vi "MOCVD_FrontPanelr.vi"() -> ()   [LabVIEW 2011]
uses:
  low_level_proc/globals.vi
panel:
  in  "Clear Log":bool
  in  "?":enum32{"Vacuum", "Heater/Spinner"}(tab)
  in  "Vac Remote":bool
  in  "Vac Exhaust":bool
  in  "Atm Exhaust":bool
  in  "Set":bool
  in  "Setpoint (C)":dbl
  in  "Heater":bool
  in  "Spinner":bool
  in  "Heater/Spinner Remote":bool
  out "Log":string
  in  "Clear All Relays":bool
  in  "Stop":bool
  in  "?":T1(tab)
  in  "display N2 or H2":bool=TRUE
  in  "N2/H2 Remote":bool
  in  "Set N2 Flow Rate":dbl min=0.0 max=1000.0
  in  "Set H2 Flow Rate":dbl min=0.0 max=1000.0
  out "H2/N2 Actual Flow Rate":dbl
  in  "N2 On":bool
  in  "H2 On":bool
  in  "Set Al Flow Rate":dbl min=0.0 max=100.0
  out "Actual Al Flow Rate":dbl
  in  "Al Remote":bool
  in  "Al Active":bool
  in  "Al Bubbler":bool
  in  "Al Run":bool
  out "GAMFC1":dbl format="%4.2g"
  out "GAMFC2":dbl format="%4.2g"
  out "GAMFC3":i16
  in  "Ga Set  Flow Rate 2 (Bubbler)":dbl min=0.0 max=10.0 format="%4.2f"
  in  "Ga Set Flow Rate 1 (Out)":dbl min=0.0 max=1.0 format="%4.2g"
  in  "Ga Active":bool
  in  "Ga Bubbler":bool
  in  "Ga Run":bool
  in  "Ga H2 Dilute":bool
  in  "Ga Remote":bool
  in  "Ga Set Flow Rate 3 (Vent)":i16 min=0 max=1000
  in  "Set In Flow Rate":dbl min=0.0 max=100.0
  out "Actual In Flow Rate":dbl
  in  "In Remote":bool
  in  "In Active":bool
  in  "In Bubbler":bool
  in  "In Run":bool
  in  "Set P_Gas Flow Rate":dbl min=0.0 max=1000.0
  out "Actual P_Gas Flow Rate":dbl
  in  "P_Gas Remote":bool
  in  "P_Gas Active":bool
  in  "P_Gas In":bool
  in  "P_Gas Run":bool
  in  "P_Gas H2 In":bool
  in  "As Gas Set Flow Rate":dbl min=0.0 max=1000.0
  out "As Gas Actual Flow Rate":dbl
  in  "As Gas Run":bool
  in  "As Gas  H2 In":bool
  in  "As Gas Active":bool
  in  "As Gas In":bool
  in  "As Gas Remote":bool
  in  "Set P_Liq Flow Rate":dbl min=0.0 max=100.0
  out "Actual P_Liq Flow Rate":dbl
  in  "P_Liq Remote":bool
  in  "P_Liq Active":bool
  in  "P_Liq Bubbler":bool
  in  "P_Liq Run":bool
  in  "Set As_Liq Flow Rate":dbl min=0.0 max=100.0
  out "Actual As_Liq Flow Rate":dbl
  in  "As_Liq Remote":bool
  in  "As_Liq Active":bool
  in  "As_Liq Bubbler":bool
  in  "As_Liq Run":bool
  out "Actual Flow Rate 1 (Out)":dbl
  out "Actual Flow Rate 2 (Bubbler)":dbl
  out "Actual Flow Rate 3 (Vent)":dbl
  in  "Fe Set Flow Rate 1 (Out)":dbl min=0.0 max=100.0
  in  "Fe SetFlow Rate 2 (Bubbler)":dbl min=0.0 max=100.0
  in  "Fe Active":bool
  in  "Fe Bubbler":bool
  in  "Fe H2 Dilute":bool
  in  "Fe Run":bool
  in  "Fe Remote":bool
  in  "Fe Set Flow Rate 3 (Vent)":dbl min=0.0 max=100.0
  in  "?":enum32{"P-Dopant", "N-Dopant"}(tab)
  in  "P_Dop Gas Source":bool
  in  "P_Dop H2 Dilute":bool
  in  "P_Dop Run":bool
  in  "P_Dop Bubbler":bool
  in  "P_Dop Active":bool
  in  "Set P Dopant Flow Rate 1":dbl min=0.0 max=100.0
  in  "Set P Dopant Flow Rate 2":dbl min=0.0 max=100.0
  in  "Set P Dopant Flow Rate 3":dbl min=0.0 max=1000.0
  in  "Set P Dopant Flow Rate 4":dbl min=0.0 max=100.0
  in  "P_Dop Remote":bool
  in  "Set N Dopant Flow Rate 1":dbl min=0.0 max=100.0
  in  "Set N Dopant Flow Rate 2":dbl min=0.0 max=100.0
  in  "Set N Dopant Flow Rate 3":dbl min=0.0 max=1000.0
  in  "Set N Dopant Flow Rate 4":dbl min=0.0 max=10.0
  in  "N_Dop Remote":bool
  in  "N_Dop Gas Source":bool
  in  "N_Dop H2 Dilute":bool
  in  "N_Dop Run":bool
  in  "N_Dop Active":bool
  in  "N_Dop Bubbler":bool
  out "Actual NP Dopant Flow Rate 1":dbl
  out "Actual NP Dopant Flow Rate 2, 4":dbl
  out "Actual N Dopant Flow Rate 3":dbl
  in  "Display N or P":bool
  in  "6940B GPIB Address":string="23"
  # "0-10000 sscm"
  # "0-10000 sscm"
  # "Display:"
  # "N2"
  # "H2"
  # "100 sscm"
  # "10 sscm"
  # "10 sscm"
  # "1000 sscm"
  # "100 sscm"
  # "100 sscm"
  # "10 sscm"
  # "100 sscm"
  # "100 sscm"
  # "100 sscm"
  # "100 sscm"
  # "1000 sscm"
  # "100 sscm"
  # "100 sscm"
  # "1000 sscm"
  # "100 sscm"
  # "100 sscm"
  # "100 sscm"
  # "1000 sscm"
  # "10 sscm"
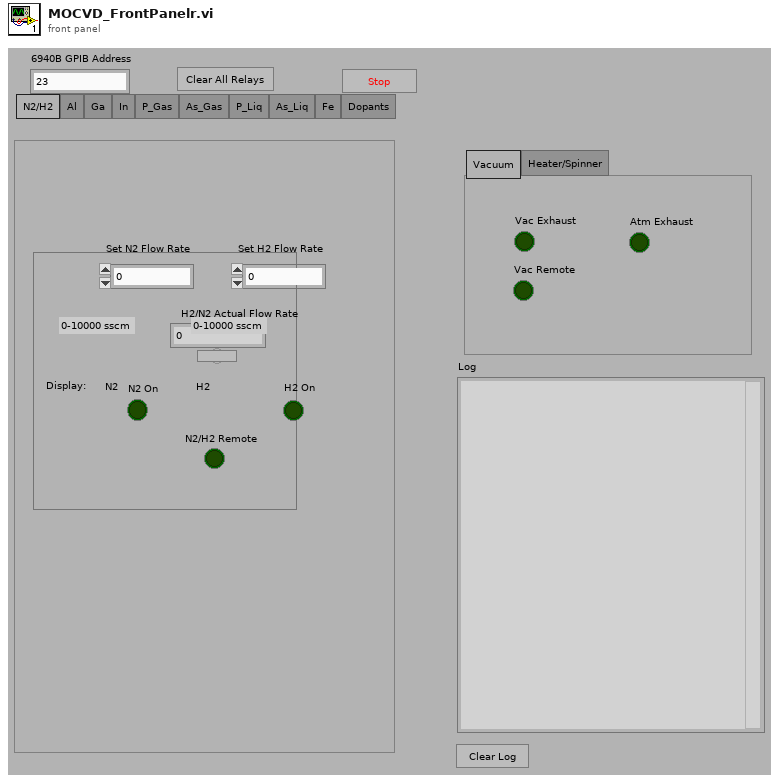
[diagram p1: front panel]
types:
  T1 = enum32{"N2/H2", "Al", "Ga", "In", "P_Gas", "As_Gas", "P_Liq", "As_Liq", "Fe", "Dopants"}
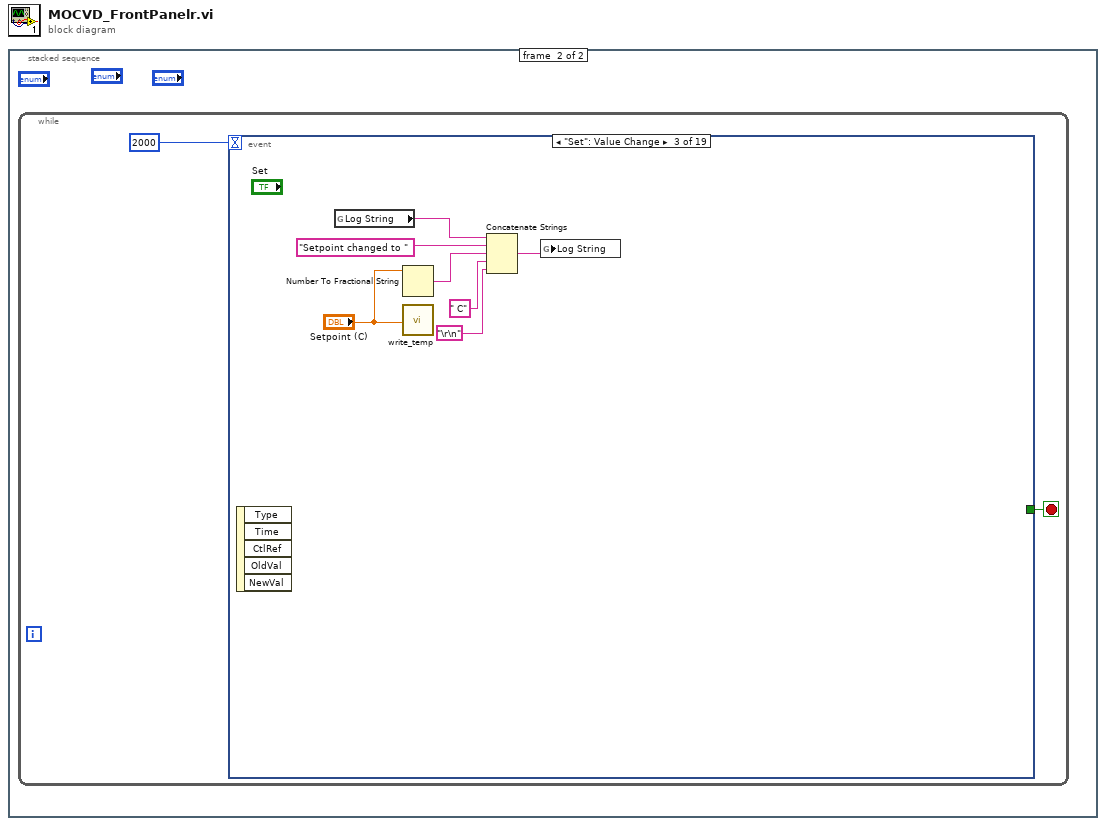
[diagram p0: block diagram]
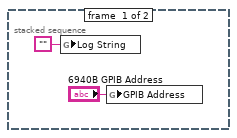
[diagram p2: hidden frame]
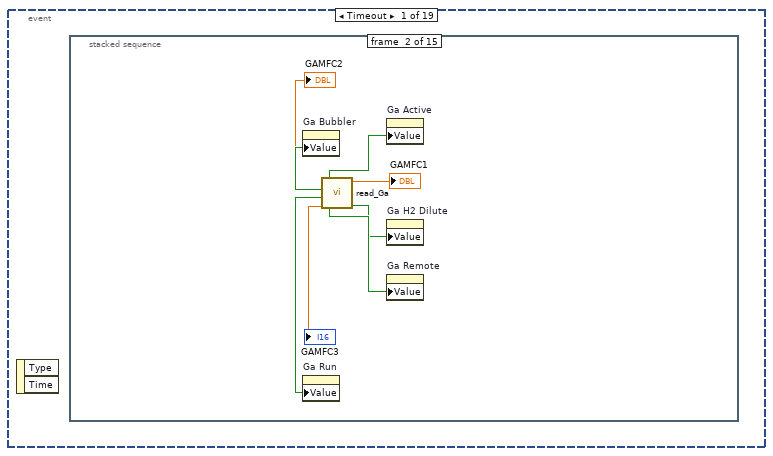
[diagram p3: hidden frame]
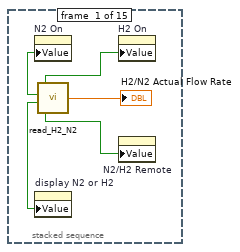
[diagram p4: hidden frame]
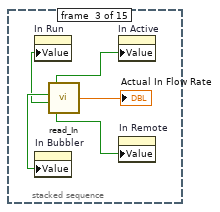
[diagram p5: hidden frame]
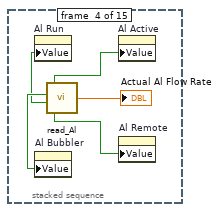
[diagram p6: hidden frame]
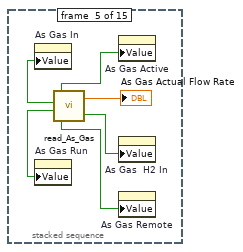
[diagram p7: hidden frame]
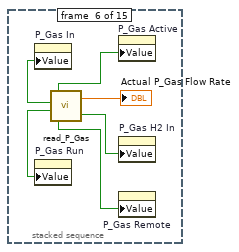
[diagram p8: hidden frame]
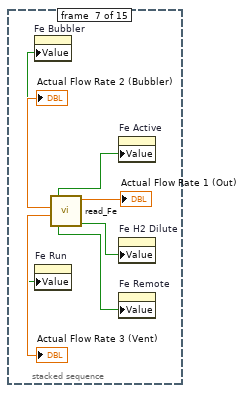
[diagram p9: hidden frame]
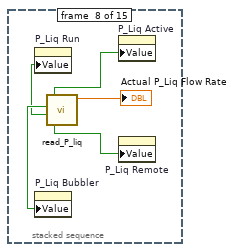
[diagram p10: hidden frame]
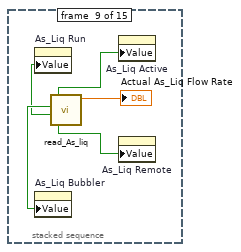
[diagram p11: hidden frame]
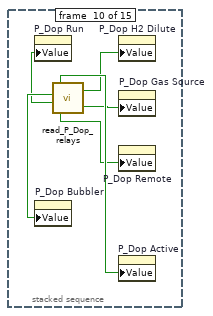
[diagram p12: hidden frame]
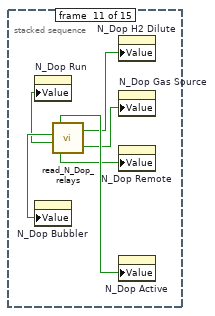
[diagram p13: hidden frame]
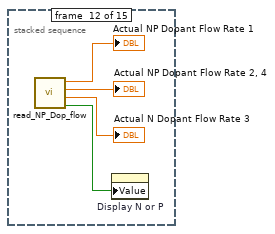
[diagram p14: hidden frame]
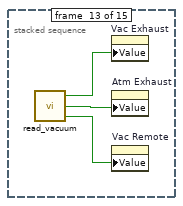
[diagram p15: hidden frame]
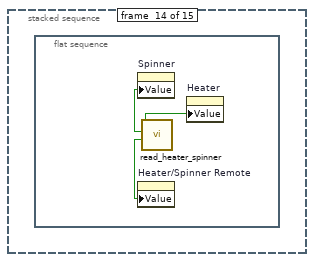
[diagram p16: hidden frame]
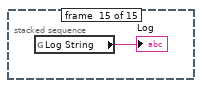
[diagram p17: hidden frame]
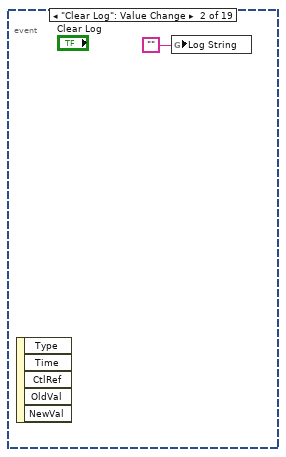
[diagram p18: hidden frame]
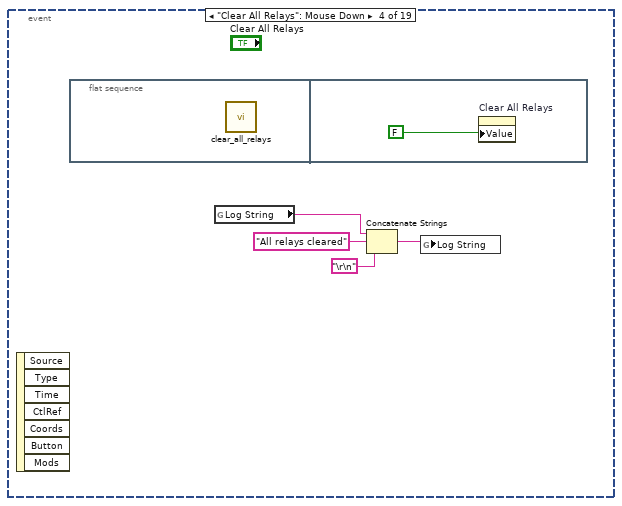
[diagram p19: hidden frame]
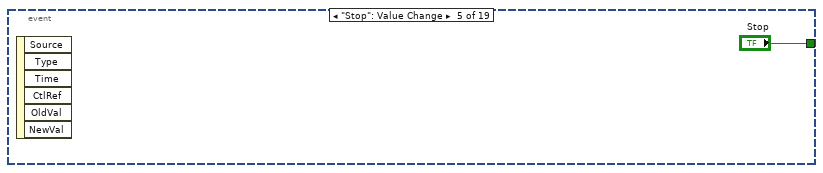
[diagram p20: hidden frame]
diagram:
  n1 = stacked-sequence {
    frame #0 {
      n2 = global write "globals.vi" "Log String"("") -> ()
      n3 = global write "globals.vi" "GPIB Address"("6940B GPIB Address") -> ()
    }
    frame #1 {
      n4 = while {
        stop <- w4 stop-if-true
        n5 = event shown="[2] \"Set\": Value Change" {
          selector: _ -> [_ _ _ _ _ _ _ _ _ _ _ _ _ _ _ _ _ _ _]
          dyn-events: _ -> [_ _ _ _ _ _ _ _ _ _ _ _ _ _ _ _ _ _ _]
          timeout: 2000 -> [_ _ _ _ _ _ _ _ _ _ _ _ _ _ _ _ _ _ _]
          tunnel: [_ _ _ _ "Stop" _ _ _ _ _ _ _ _ _ _ _ _ _ _] -> w4
          event Timeout {
            n6 = event-data() -> ()  [unwired: 3 out]
            n7 = stacked-sequence {
              frame #0 {
                n8 = call "read_H2_N2.vi"() -> ("H2N2 Flow Rate"=→"H2/N2 Actual Flow Rate":dbl, "H2N2 Remote"=w9:bool, "Display H2N2"=w8:bool, "N2 Active"=w7:bool, "H2 Active"=w6:bool)
                n9 = property on="N2 On" class="Bool (strict)"("Value"=w7) -> ()  [unwired: 2 in, 2 out]
                n10 = property on="display N2 or H2" class="Bool (strict)"("Value"=w8) -> ()  [unwired: 2 in, 2 out]
                n11 = property on="H2 On" class="Bool (strict)"("Value"=w6) -> ()  [unwired: 2 in, 2 out]
                n12 = property on="N2/H2 Remote" class="Bool (strict)"("Value"=w9) -> ()  [unwired: 2 in, 2 out]
              }
              frame #1 {
                n13 = call "read_Ga.vi"() -> ("H2 Dilute"=w13:bool, "GAMFC3"=→"GAMFC3":dbl, "GAMFC2"=→"GAMFC2":dbl, "GAMFC1"=→"GAMFC1":dbl, "Ga Remote"=w16:bool, "Ga Run"=w17:bool, "Ga Bubbler"=w14:bool, "Ga Active"=w15:bool)
                n14 = property on="Ga Bubbler" class="Bool (strict)"("Value"=w14) -> ()  [unwired: 2 in, 2 out]
                n15 = property on="Ga Run" class="Bool (strict)"("Value"=w17) -> ()  [unwired: 2 in, 2 out]
                n16 = property on="Ga Active" class="Bool (strict)"("Value"=w15) -> ()  [unwired: 2 in, 2 out]
                n17 = property on="Ga H2 Dilute" class="Bool (strict)"("Value"=w13) -> ()  [unwired: 2 in, 2 out]
                n18 = property on="Ga Remote" class="Bool (strict)"("Value"=w16) -> ()  [unwired: 2 in, 2 out]
              }
              frame #2 {
                n19 = call "read_In.vi"() -> ("Actual In Flow Rate"=→"Actual In Flow Rate":dbl, "In Remote"=w19:bool, "In Run"=w18:bool, "In Bubbler"=w20:bool, "In Active"=w21:bool)
                n20 = property on="In Run" class="Bool (strict)"("Value"=w18) -> ()  [unwired: 2 in, 2 out]
                n21 = property on="In Bubbler" class="Bool (strict)"("Value"=w20) -> ()  [unwired: 2 in, 2 out]
                n22 = property on="In Active" class="Bool (strict)"("Value"=w21) -> ()  [unwired: 2 in, 2 out]
                n23 = property on="In Remote" class="Bool (strict)"("Value"=w19) -> ()  [unwired: 2 in, 2 out]
              }
              frame #3 {
                n24 = call "read_Al.vi"() -> ("Actual Al Flow Rate"=→"Actual Al Flow Rate":dbl, "Al Remote"=w23:bool, "Al Run"=w25:bool, "Al Bubbler"=w26:bool, "Al Active"=w27:bool)
                n25 = property on="Al Run" class="Bool (strict)"("Value"=w25) -> ()  [unwired: 2 in, 2 out]
                n26 = property on="Al Bubbler" class="Bool (strict)"("Value"=w26) -> ()  [unwired: 2 in, 2 out]
                n27 = property on="Al Active" class="Bool (strict)"("Value"=w27) -> ()  [unwired: 2 in, 2 out]
                n28 = property on="Al Remote" class="Bool (strict)"("Value"=w23) -> ()  [unwired: 2 in, 2 out]
              }
              frame #4 {
                n29 = call "read_As_Gas.vi"() -> ("As Gas H2 In"=w28:bool, "As Gas Actual Flow Rate"=→"As Gas Actual Flow Rate":dbl, "As Gas Remote"=w32:bool, "As Gas Run"=w31:bool, "As Gas In"=w30:bool, "As Gas Active"=w29:bool)
                n30 = property on="As Gas In" class="Bool (strict)"("Value"=w30) -> ()  [unwired: 2 in, 2 out]
                n31 = property on="As Gas Run" class="Bool (strict)"("Value"=w31) -> ()  [unwired: 2 in, 2 out]
                n32 = property on="As Gas Active" class="Bool (strict)"("Value"=w29) -> ()  [unwired: 2 in, 2 out]
                n33 = property on="As Gas  H2 In" class="Bool (strict)"("Value"=w28) -> ()  [unwired: 2 in, 2 out]
                n34 = property on="As Gas Remote" class="Bool (strict)"("Value"=w32) -> ()  [unwired: 2 in, 2 out]
              }
              frame #5 {
                n35 = call "read_P_Gas.vi"() -> ("P Gas H2 In"=w34:bool, "P Gas Actual Flow Rate"=→"Actual P_Gas Flow Rate":dbl, "P Gas Remote"=w38:bool, "P Gas Run"=w37:bool, "P Gas In"=w36:bool, "P Gas Active"=w35:bool)
                n36 = property on="P_Gas In" class="Bool (strict)"("Value"=w36) -> ()  [unwired: 2 in, 2 out]
                n37 = property on="P_Gas Run" class="Bool (strict)"("Value"=w37) -> ()  [unwired: 2 in, 2 out]
                n38 = property on="P_Gas Active" class="Bool (strict)"("Value"=w35) -> ()  [unwired: 2 in, 2 out]
                n39 = property on="P_Gas H2 In" class="Bool (strict)"("Value"=w34) -> ()  [unwired: 2 in, 2 out]
                n40 = property on="P_Gas Remote" class="Bool (strict)"("Value"=w38) -> ()  [unwired: 2 in, 2 out]
              }
              frame #6 {
                n41 = call "read_Fe.vi"() -> ("Fe H2 Dilute"=w44:bool, "Actual Fe Flow Rate 3 (Vent)"=→"Actual Flow Rate 3 (Vent)":dbl, "Actual Fe Flow Rate2 (Bubbler)"=→"Actual Flow Rate 2 (Bubbler)":dbl, "Actual Fe Flow Rate1  (Out)"=→"Actual Flow Rate 1 (Out)":dbl, "Fe Remote"=w43:bool, "Fe Run"=w42:bool, "Fe Bubbler"=w41:bool, "Fe Active"=w40:bool)
                n42 = property on="Fe Bubbler" class="Bool (strict)"("Value"=w41) -> ()  [unwired: 2 in, 2 out]
                n43 = property on="Fe Run" class="Bool (strict)"("Value"=w42) -> ()  [unwired: 2 in, 2 out]
                n44 = property on="Fe Active" class="Bool (strict)"("Value"=w40) -> ()  [unwired: 2 in, 2 out]
                n45 = property on="Fe H2 Dilute" class="Bool (strict)"("Value"=w44) -> ()  [unwired: 2 in, 2 out]
                n46 = property on="Fe Remote" class="Bool (strict)"("Value"=w43) -> ()  [unwired: 2 in, 2 out]
              }
              frame #7 {
                n47 = call "read_P_liq.vi"() -> ("Actual P liq Flow Rate"=→"Actual P_Liq Flow Rate":dbl, "P liq Remote"=w49:bool, "P liq Run"=w48:bool, "P liq Bubbler"=w51:bool, "P liq Active"=w50:bool)  [unwired: 3 out]
                n48 = property on="P_Liq Run" class="Bool (strict)"("Value"=w48) -> ()  [unwired: 2 in, 2 out]
                n49 = property on="P_Liq Bubbler" class="Bool (strict)"("Value"=w51) -> ()  [unwired: 2 in, 2 out]
                n50 = property on="P_Liq Active" class="Bool (strict)"("Value"=w50) -> ()  [unwired: 2 in, 2 out]
                n51 = property on="P_Liq Remote" class="Bool (strict)"("Value"=w49) -> ()  [unwired: 2 in, 2 out]
              }
              frame #8 {
                n52 = call "read_As_liq.vi"() -> ("Actual As liq Flow Rate"=→"Actual As_Liq Flow Rate":dbl, "As liq Remote"=w53:bool, "As liq Run"=w54:bool, "As liq Bubbler"=w55:bool, "As liq Active"=w56:bool)  [unwired: 3 out]
                n53 = property on="As_Liq Run" class="Bool (strict)"("Value"=w54) -> ()  [unwired: 2 in, 2 out]
                n54 = property on="As_Liq Bubbler" class="Bool (strict)"("Value"=w55) -> ()  [unwired: 2 in, 2 out]
                n55 = property on="As_Liq Active" class="Bool (strict)"("Value"=w56) -> ()  [unwired: 2 in, 2 out]
                n56 = property on="As_Liq Remote" class="Bool (strict)"("Value"=w53) -> ()  [unwired: 2 in, 2 out]
              }
              frame #9 {
                n57 = call "read_P_Dop_relays.vi"() -> ("P_Dop Gas Source"=w60:bool, "P_Dop H2 Dilute"=w61:bool, "P_Dop Remote"=w58:bool, "P_Dop Run"=w59:bool, "P_Dop Bubbler"=w62:bool, "P_Dop Active"=w63:bool)
                n58 = property on="P_Dop Run" class="Bool (strict)"("Value"=w59) -> ()  [unwired: 2 in, 2 out]
                n59 = property on="P_Dop Bubbler" class="Bool (strict)"("Value"=w62) -> ()  [unwired: 2 in, 2 out]
                n60 = property on="P_Dop H2 Dilute" class="Bool (strict)"("Value"=w61) -> ()  [unwired: 2 in, 2 out]
                n61 = property on="P_Dop Gas Source" class="Bool (strict)"("Value"=w60) -> ()  [unwired: 2 in, 2 out]
                n62 = property on="P_Dop Remote" class="Bool (strict)"("Value"=w58) -> ()  [unwired: 2 in, 2 out]
                n63 = property on="P_Dop Active" class="Bool (strict)"("Value"=w63) -> ()  [unwired: 2 in, 2 out]
              }
              frame #10 {
                n64 = call "read_N_Dop_relays.vi"() -> ("N_Dop Gas Source"=w64:bool, "N_Dop H2 Dilute"=w65:bool, "N_Dop Remote"=w66:bool, "N_Dop Run"=w67:bool, "N_Dop Bubbler"=w68:bool, "N_Dop Active"=w69:bool)
                n65 = property on="N_Dop Run" class="Bool (strict)"("Value"=w67) -> ()  [unwired: 2 in, 2 out]
                n66 = property on="N_Dop Bubbler" class="Bool (strict)"("Value"=w68) -> ()  [unwired: 2 in, 2 out]
                n67 = property on="N_Dop H2 Dilute" class="Bool (strict)"("Value"=w65) -> ()  [unwired: 2 in, 2 out]
                n68 = property on="N_Dop Gas Source" class="Bool (strict)"("Value"=w64) -> ()  [unwired: 2 in, 2 out]
                n69 = property on="N_Dop Remote" class="Bool (strict)"("Value"=w66) -> ()  [unwired: 2 in, 2 out]
                n70 = property on="N_Dop Active" class="Bool (strict)"("Value"=w69) -> ()  [unwired: 2 in, 2 out]
              }
              frame #11 {
                n71 = call "read_NP_Dop_flow.vi"() -> ("N/P Dopant DA Switch"=w73:bool, "N/P_Dop Flow 3"=→"Actual N Dopant Flow Rate 3":dbl, "N/P_Dop Flow 2 or 4"=→"Actual NP Dopant Flow Rate 2, 4":dbl, "N/P_Dop Flow 1"=→"Actual NP Dopant Flow Rate 1":dbl)
                n72 = property on="Display N or P" class="Bool (strict)"("Value"=w73) -> ()  [unwired: 2 in, 2 out]
              }
              frame #12 {
                n73 = call "read_vacuum.vi"() -> ("Vac Remote"=w76:bool, "Atm Exhaust"=w75:bool, "Vac Exhaust"=w74:bool)
                n74 = property on="Vac Exhaust" class="Bool (strict)"("Value"=w74) -> ()  [unwired: 2 in, 2 out]
                n75 = property on="Atm Exhaust" class="Bool (strict)"("Value"=w75) -> ()  [unwired: 2 in, 2 out]
                n76 = property on="Vac Remote" class="Bool (strict)"("Value"=w76) -> ()  [unwired: 2 in, 2 out]
              }
              frame #13 {
                n77 = flat-sequence {
                  frame #0 {
                    n78 = call "read_heater_spinner.vi"() -> ("Heater/Spinner Remote"=w77:bool, "Spinner"=w78:bool, "Heater"=w79:bool)  [unwired: 7 out]
                    n79 = property on="Spinner" class="Bool (strict)"("Value"=w78) -> ()  [unwired: 2 in, 2 out]
                    n80 = property on="Heater/Spinner Remote" class="Bool (strict)"("Value"=w77) -> ()  [unwired: 2 in, 2 out]
                    n81 = property on="Heater" class="Bool (strict)"("Value"=w79) -> ()  [unwired: 2 in, 2 out]
                  }
                }
              }
              frame #14 {
                n82 = global read "globals.vi" "Log String"() -> (→"Log":string)
              }
            }
          }
          event "Clear Log": Value Change {
            n83 = event-data() -> ()  [unwired: 6 out]
            n84 = global write "globals.vi" "Log String"("") -> ()
          }
          event "Set": Value Change {
            n85 = event-data() -> ()  [unwired: 6 out]
            n86 = global read "globals.vi" "Log String"() -> (w87:string)
            n87 = Number To Fractional String(number="Setpoint (C)") -> (F-format string=w86:string)  [unwired: 3 in]
            n88 = call "write_temp.vi"("Temperature (C)"="Setpoint (C)") -> ()  [unwired: 1 out]
            n89 = Concatenate Strings(w87, "Setpoint changed to " ("string"), w86, " C" ("string"), "\r\n") -> (w88:string)
            n90 = global write "globals.vi" "Log String"(w88) -> ()
          }
          event "Clear All Relays": Mouse Down {
            n91 = event-data() -> ()  [unwired: 8 out]
            n92 = flat-sequence {
              frame #0 {
                n93 = call "clear_all_relays.vi"() -> ()  [unwired: 2 out]
              }
              frame #1 {
                n94 = property on="Clear All Relays" class="Bool (strict)"("Value"=FALSE ("Clear All Relays")) -> ()  [unwired: 2 in, 2 out]
              }
            }
            n95 = global read "globals.vi" "Log String"() -> (w91:string)
            n96 = Concatenate Strings(w91, "All relays cleared" ("string"), "\r\n") -> (w92:string)
            n97 = global write "globals.vi" "Log String"(w92) -> ()
          }
          event "Stop": Value Change {
            n98 = event-data() -> ()  [unwired: 7 out]
          }
          event "N2/H2 Remote", "display N2 or H2", "N2 On", "H2 On", "Set N2 Flow Rate", "Set H2 Flow Rate": Value Change {
            n99 = event-data() -> ()  [unwired: 7 out]
            n100 = call "set_N2.vi"("Manifold N2 Flow"="Set N2 Flow Rate", "Display H2 or N2"="display N2 or H2", "N2 Active"="N2 On", "H2N2 Remote"="N2/H2 Remote") -> ()  [unwired: 2 out]
            n101 = call "set_H2.vi"("Manifold H2 Flow"="Set H2 Flow Rate", "Display H2 or N2"="display N2 or H2", "H2 Active"="H2 On", "H2N2 Remote"="N2/H2 Remote") -> ()  [unwired: 2 in]
            n102 = global read "globals.vi" "Log String"() -> (w118:string)
            n103 = Number To Fractional String(number="Set N2 Flow Rate") -> (F-format string=w104:string)  [unwired: 3 in]
            n104 = Number To Fractional String(number="Set H2 Flow Rate") -> (F-format string=w100:string)  [unwired: 3 in]
            n105 = Select(t="N2 On ", s="N2 On", f="") -> (s? t:f=w114:string)
            n106 = Select(t="H2 On ", s="H2 On", f="") -> (s? t:f=w110:string)
            n107 = Select(t="N2/H2 Remote ", s="N2/H2 Remote", f="") -> (s? t:f=w106:string)
            n108 = Concatenate Strings("N2 Rate " ("string"), w104, " " ("string")) -> (w101:string)
            n109 = Concatenate Strings("H2 Rate " ("string"), w100, " " ("string")) -> (w96:string)
            n110 = Concatenate Strings(w118, w114, w110, w106, w101, w96, "\r\n") -> (w119:string)
            n111 = global write "globals.vi" "Log String"(w119) -> ()
          }
          event "In Remote", "In Active", "In Bubbler", "In Run", "Set In Flow Rate": Value Change {
            n112 = event-data() -> ()  [unwired: 7 out]
            n113 = call "set_In.vi"("Indium Flow"="Set In Flow Rate", "In Remote"="In Remote", "In Run"="In Run", "In Bubbler"="In Bubbler", "In Active"="In Active") -> ()  [unwired: 5 out]
            n114 = Number To Fractional String(number="Set In Flow Rate") -> (F-format string=w143:string)  [unwired: 3 in]
            n115 = Concatenate Strings("In Rate " ("string"), w143, " " ("string")) -> (w139:string)
            n116 = Select(t="In Active ", s="In Active", f="") -> (s? t:f=w126:string)
            n117 = Select(t="In Bubbler ", s="In Bubbler", f="") -> (s? t:f=w125:string)
            n118 = Select(t="In Run ", s="In Run", f="") -> (s? t:f=w124:string)
            n119 = Select(t="In Remote ", s="In Remote", f="") -> (s? t:f=w123:string)
            n120 = global read "globals.vi" "Log String"() -> (w140:string)
            n121 = Concatenate Strings(w140, w139, w126, w125, w124, w123, "\r\n") -> (w122:string)
            n122 = global write "globals.vi" "Log String"(w122) -> ()
          }
          event "Al Remote", "Al Active", "Al Bubbler", "Al Run", "Set Al Flow Rate": Value Change {
            n123 = event-data() -> ()  [unwired: 7 out]
            n124 = call "set_Al.vi"("Aluminum Flow"="Set Al Flow Rate", "Al Remote"="Al Remote", "Al Run"="Al Run", "Al Bubbler"="Al Bubbler", "Al Active"="Al Active") -> ()  [unwired: 5 out]
            n125 = Number To Fractional String(number="Set Al Flow Rate") -> (F-format string=w167:string)  [unwired: 3 in]
            n126 = Concatenate Strings("Al Rate " ("string"), w167, " " ("string")) -> (w151:string)
            n127 = Select(t="Al Active ", s="Al Active", f="") -> (s? t:f=w150:string)
            n128 = Select(t="Al Bubbler ", s="Al Bubbler", f="") -> (s? t:f=w149:string)
            n129 = Select(t="Al Run ", s="Al Run", f="") -> (s? t:f=w148:string)
            n130 = Select(t="Al Remote ", s="Al Remote", f="") -> (s? t:f=w147:string)
            n131 = global read "globals.vi" "Log String"() -> (w152:string)
            n132 = Concatenate Strings(w152, w151, w150, w149, w148, w147, "\r\n") -> (w145:string)
            n133 = global write "globals.vi" "Log String"(w145) -> ()
          }
          event "P_Liq Remote", "P_Liq Active", "P_Liq Bubbler", "P_Liq Run", "Set P_Liq Flow Rate": Value Change {
            n134 = event-data() -> ()  [unwired: 7 out]
            n135 = call "set_P_Liq.vi"("P_Liq Flow"="Set P_Liq Flow Rate", "P_Liq Remote"="P_Liq Remote", "P_Liq Run"="P_Liq Run", "P_Liq Bubbler"="P_Liq Bubbler", "P_Liq Active"="P_Liq Active") -> ()  [unwired: 7 out]
            n136 = Number To Fractional String(number="Set P_Liq Flow Rate") -> (F-format string=w190:string)  [unwired: 3 in]
            n137 = Concatenate Strings("P_Liq Rate " ("string"), w190, " " ("string")) -> (w187:string)
            n138 = global read "globals.vi" "Log String"() -> (w188:string)
            n139 = Select(t="P_Liq Active ", s="P_Liq Active", f="") -> (s? t:f=w173:string)
            n140 = Select(t="P_Liq Bubbler ", s="P_Liq Bubbler", f="") -> (s? t:f=w172:string)
            n141 = Select(t="P_Liq Run ", s="P_Liq Run", f="") -> (s? t:f=w171:string)
            n142 = Select(t="P_Liq Remote ", s="P_Liq Remote", f="") -> (s? t:f=w170:string)
            n143 = Concatenate Strings(w188, w187, w173, w172, w171, w170, "\r\n") -> (w186:string)
            n144 = global write "globals.vi" "Log String"(w186) -> ()
          }
          event "As_Liq Remote", "As_Liq Active", "As_Liq Bubbler", "As_Liq Run", "Set As_Liq Flow Rate": Value Change {
            n145 = event-data() -> ()  [unwired: 7 out]
            n146 = call "set_As_Liq.vi"("As_Liq Flow"="Set As_Liq Flow Rate", "As_Liq Remote"="As_Liq Remote", "As_Liq Run"="As_Liq Run", "As_Liq Bubbler"="As_Liq Bubbler", "As_Liq Active"="As_Liq Active") -> ()  [unwired: 7 out]
            n147 = Number To Fractional String(number="Set As_Liq Flow Rate") -> (F-format string=w214:string)  [unwired: 3 in]
            n148 = Concatenate Strings("As_Liq Rate " ("string"), w214, " " ("string")) -> (w199:string)
            n149 = Select(t="As_Liq Active ", s="As_Liq Active", f="") -> (s? t:f=w198:string)
            n150 = Select(t="As_Liq Bubbler ", s="As_Liq Bubbler", f="") -> (s? t:f=w197:string)
            n151 = Select(t="As_Liq Run ", s="As_Liq Run", f="") -> (s? t:f=w196:string)
            n152 = Select(t="As_Liq Remote ", s="As_Liq Remote", f="") -> (s? t:f=w195:string)
            n153 = global read "globals.vi" "Log String"() -> (w200:string)
            n154 = Concatenate Strings(w200, w199, w198, w197, w196, w195, "\r\n") -> (w193:string)
            n155 = global write "globals.vi" "Log String"(w193) -> ()
          }
          event "P_Gas Remote", "P_Gas Active", "P_Gas In", "P_Gas Run", "P_Gas H2 In", "Set P_Gas Flow Rate": Value Change {
            n156 = event-data() -> ()  [unwired: 7 out]
            n157 = call "set_P_gas.vi"("P_Gas Active"="P_Gas Active", "P_Gas Flow"="Set P_Gas Flow Rate", "P_Gas In"="P_Gas In", "P_Gas H2 In"="P_Gas H2 In", "P_Gas Run"="P_Gas Run", "P_Gas Remote"="P_Gas Remote") -> ()  [unwired: 10 out]
            n158 = Number To Fractional String(number="Set P_Gas Flow Rate") -> (F-format string=w242:string)  [unwired: 3 in]
            n159 = Concatenate Strings("P_Gas Rate " ("string"), w242, " " ("string")) -> (w224:string)
            n160 = Select(t="P_Gas Active ", s="P_Gas Active", f="") -> (s? t:f=w223:string)
            n161 = Select(t="P_Gas In ", s="P_Gas In", f="") -> (s? t:f=w222:string)
            n162 = Select(t="P_Gas H2 In ", s="P_Gas H2 In", f="") -> (s? t:f=w221:string)
            n163 = Select(t="P_Gas Remote ", s="P_Gas Remote", f="") -> (s? t:f=w219:string)
            n164 = Select(t="P_Gas Run ", s="P_Gas Run", f="") -> (s? t:f=w220:string)
            n165 = global read "globals.vi" "Log String"() -> (w225:string)
            n166 = Concatenate Strings(w225, w224, w223, w222, w221, w220, w219, "\r\n") -> (w217:string)
            n167 = global write "globals.vi" "Log String"(w217) -> ()
          }
          event "As Gas Remote", "As Gas Run", "As Gas  H2 In", "As Gas In", "As Gas Active", "As Gas Set Flow Rate": Value Change {
            n168 = event-data() -> ()  [unwired: 7 out]
            n169 = call "set_As_gas.vi"("As_Gas Active"="As Gas Active", "As_Gas Flow"="As Gas Set Flow Rate", "As_Gas In"="As Gas In", "As_Gas H2"="As Gas  H2 In", "As_Gas Run"="As Gas Run", "As_Gas Remote"="As Gas Remote") -> ()  [unwired: 10 out]
            n170 = Number To Fractional String(number="As Gas Set Flow Rate") -> (F-format string=w271:string)  [unwired: 3 in]
            n171 = Concatenate Strings("As Gas Rate " ("string"), w271, " " ("string")) -> (w251:string)
            n172 = Select(t="As Gas In ", s="As Gas In", f="") -> (s? t:f=w249:string)
            n173 = Select(t="As Gas Active ", s="As Gas Active", f="") -> (s? t:f=w250:string)
            n174 = Select(t="As Gas H2 In ", s="As Gas  H2 In", f="") -> (s? t:f=w248:string)
            n175 = Select(t="As Gas Run ", s="As Gas Run", f="") -> (s? t:f=w247:string)
            n176 = Select(t="As Gas Remote ", s="As Gas Remote", f="") -> (s? t:f=w246:string)
            n177 = global read "globals.vi" "Log String"() -> (w253:string)
            n178 = Concatenate Strings(w253, w251, w250, w249, w248, w247, w246, "\r\n") -> (w252:string)
            n179 = global write "globals.vi" "Log String"(w252) -> ()
          }
          event "Ga Active", "Ga Bubbler", "Ga Run", "Ga Set Flow Rate 1 (Out)", "Ga Set  Flow Rate 2 (Bubbler)", "Ga Set Flow Rate 3 (Vent)", "Ga Remote", "Ga H2 Dilute": Value Change {
            n180 = event-data() -> ()  [unwired: 6 out]
            n181 = call "set_Ga.vi"("Ga Active"="Ga Active", "Ga Flow 3"="Ga Set Flow Rate 3 (Vent)", "Ga Flow 2"="Ga Set  Flow Rate 2 (Bubbler)", "Ga Flow 1"="Ga Set Flow Rate 1 (Out)", "Ga Bubbler"="Ga Bubbler", "Ga H2 Dilute"="Ga H2 Dilute", "Ga Run"="Ga Run", "Ga Remote"="Ga Remote") -> ()  [unwired: 8 out]
            n182 = Number To Fractional String(number="Ga Set  Flow Rate 2 (Bubbler)") -> (F-format string=w306:string)  [unwired: 3 in]
            n183 = Number To Fractional String(number="Ga Set Flow Rate 1 (Out)") -> (F-format string=w309:string)  [unwired: 3 in]
            n184 = Number To Fractional String(number="Ga Set Flow Rate 3 (Vent)") -> (F-format string=w302:string)  [unwired: 3 in]
            n185 = Concatenate Strings("Ga Rate 2 " ("string"), w306, " " ("string")) -> (w281:string)
            n186 = Select(t="Ga Active ", s="Ga Active", f="") -> (s? t:f=w279:string)
            n187 = Concatenate Strings("Ga Rate 1 " ("string"), w309, " " ("string")) -> (w282:string)
            n188 = Select(t="Ga Bubbler ", s="Ga Bubbler", f="") -> (s? t:f=w278:string)
            n189 = Concatenate Strings("Ga Rate 3 " ("string"), w302, " " ("string")) -> (w280:string)
            n190 = Select(t="Ga H2 Dilute ", s="Ga H2 Dilute", f="") -> (s? t:f=w277:string)
            n191 = Select(t="Ga Run ", s="Ga Run", f="") -> (s? t:f=w276:string)
            n192 = Select(t="Ga Remote ", s="Ga Remote", f="") -> (s? t:f=w275:string)
            n193 = global read "globals.vi" "Log String"() -> (w283:string)
            n194 = Concatenate Strings(w283, w282, w281, w280, w279, w278, w277, w276, w275, "\r\n") -> (w273:string)
            n195 = global write "globals.vi" "Log String"(w273) -> ()
          }
          event "Fe Active", "Fe Bubbler", "Fe Run", "Fe H2 Dilute", "Fe Remote", "Fe Set Flow Rate 1 (Out)", "Fe SetFlow Rate 2 (Bubbler)": Value Change {
            n196 = event-data() -> ()  [unwired: 7 out]
            n197 = call "set_Fe.vi"("Active"="Fe Active", "Fe Flow 3"="Fe Set Flow Rate 3 (Vent)", "Fe Flow 2"="Fe SetFlow Rate 2 (Bubbler)", "Fe Flow 1"="Fe Set Flow Rate 1 (Out)", "Bubbler"="Fe Bubbler", "H2 Dilute"="Fe H2 Dilute", "Run"="Fe Run", "Remote"="Fe Remote") -> ()  [unwired: 8 out]
            n198 = Number To Fractional String(number="Fe SetFlow Rate 2 (Bubbler)") -> (F-format string=w345:string)  [unwired: 3 in]
            n199 = Number To Fractional String(number="Fe Set Flow Rate 1 (Out)") -> (F-format string=w348:string)  [unwired: 3 in]
            n200 = Number To Fractional String(number="Fe Set Flow Rate 3 (Vent)") -> (F-format string=w342:string)  [unwired: 3 in]
            n201 = Concatenate Strings("Fe Rate 2 " ("string"), w345, " " ("string")) -> (w327:string)
            n202 = Select(t="Fe Active ", s="Fe Active", f="") -> (s? t:f=w325:string)
            n203 = Concatenate Strings("Fe Rate 1 " ("string"), w348, " " ("string")) -> (w328:string)
            n204 = Select(t="Fe Bubbler ", s="Fe Bubbler", f="") -> (s? t:f=w324:string)
            n205 = Concatenate Strings("Fe Rate 3 " ("string"), w342, " " ("string")) -> (w326:string)
            n206 = Select(t="Fe H2 Dilute ", s="Fe H2 Dilute", f="") -> (s? t:f=w323:string)
            n207 = Select(t="Fe Run ", s="Fe Run", f="") -> (s? t:f=w322:string)
            n208 = Select(t="Fe Remote ", s="Fe Remote", f="") -> (s? t:f=w321:string)
            n209 = global read "globals.vi" "Log String"() -> (w329:string)
            n210 = Concatenate Strings(w329, w328, w327, w326, w325, w324, w323, w322, w321, "\r\n") -> (w319:string)
            n211 = global write "globals.vi" "Log String"(w319) -> ()
          }
          event "Heater", "Spinner", "Heater/Spinner Remote": Value Change {
            n212 = event-data() -> ()  [unwired: 7 out]
            n213 = call "set_heater_spinner.vi"("Heater/Spinner Remote"="Heater/Spinner Remote", "Spinner"="Spinner", "Heater"="Heater") -> ()  [unwired: 7 out]
            n214 = Select(t="Heater ", s="Heater", f="") -> (s? t:f=w353:string)
            n215 = Select(t="Spinner ", s="Spinner", f="") -> (s? t:f=w352:string)
            n216 = Select(t="Heater/Spinner Remote ", s="Heater/Spinner Remote", f="") -> (s? t:f=w351:string)
            n217 = global read "globals.vi" "Log String"() -> (w354:string)
            n218 = Concatenate Strings(w354, w353, w352, w351, "\r\n") -> (w349:string)
            n219 = global write "globals.vi" "Log String"(w349) -> ()
          }
          event "P_Dop Remote", "P_Dop Active", "P_Dop Bubbler", "P_Dop Run", "P_Dop H2 Dilute", "P_Dop Gas Source", "Set P Dopant Flow Rate 1", "Set P Dopant Flow Rate 2", "Set P Dopant Flow Rate 3", "Set P Dopant Flow Rate 4": Value Change {
            n220 = event-data() -> ()  [unwired: 7 out]
            n221 = call "set_P_Dop.vi"("P_Dop Active"="P_Dop Active", "P_Dop Bubbler"="P_Dop Bubbler", "P_Dop H2 Dilute"="P_Dop H2 Dilute", "P_Dop Gas Source"="P_Dop Gas Source", "P_Dop Run"="P_Dop Run", "P_Dop Remote"="P_Dop Remote", "P_Dop Flow 4"="Set P Dopant Flow Rate 4", "P_Dop Flow 3"="Set P Dopant Flow Rate 3", "P_Dop Flow 2"="Set P Dopant Flow Rate 2", "P_Dop Flow 1"="Set P Dopant Flow Rate 1") -> ()  [unwired: 10 out]
            n222 = Number To Fractional String(number="Set P Dopant Flow Rate 2") -> (F-format string=w403:string)  [unwired: 3 in]
            n223 = Number To Fractional String(number="Set P Dopant Flow Rate 4") -> (F-format string=w375:string)  [unwired: 3 in]
            n224 = Number To Fractional String(number="Set P Dopant Flow Rate 1") -> (F-format string=w406:string)  [unwired: 3 in]
            n225 = Number To Fractional String(number="Set P Dopant Flow Rate 3") -> (F-format string=w400:string)  [unwired: 3 in]
            n226 = Select(t="P_Dop Active ", s="P_Dop Active", f="") -> (s? t:f=w383:string)
            n227 = Concatenate Strings("P_Dop Rate 2 " ("string"), w403, " " ("string")) -> (w385:string)
            n228 = Concatenate Strings("P_Dop Rate 4 " ("string"), w375, " " ("string")) -> (w374:string)
            n229 = Select(t="P_Dop Bubbler ", s="P_Dop Bubbler", f="") -> (s? t:f=w382:string)
            n230 = Concatenate Strings("P_Dop Rate 1 " ("string"), w406, " " ("string")) -> (w386:string)
            n231 = Select(t="P_Dop H2 Dilute ", s="P_Dop H2 Dilute", f="") -> (s? t:f=w381:string)
            n232 = Select(t="P_Dop Run ", s="P_Dop Run", f="") -> (s? t:f=w380:string)
            n233 = Select(t="P_Dop Remote ", s="P_Dop Remote", f="") -> (s? t:f=w379:string)
            n234 = Concatenate Strings("P_Dop Rate 3 " ("string"), w400, " " ("string")) -> (w384:string)
            n235 = global read "globals.vi" "Log String"() -> (w387:string)
            n236 = Concatenate Strings(w387, w386, w385, w384, w374, w383, w382, w381, w380, w379, "\r\n") -> (w377:string)
            n237 = global write "globals.vi" "Log String"(w377) -> ()
          }
          event "N_Dop H2 Dilute", "N_Dop Bubbler", "N_Dop Run", "Set N Dopant Flow Rate 1", "Set N Dopant Flow Rate 2", "Set N Dopant Flow Rate 3", "Set N Dopant Flow Rate 4", "N_Dop Gas Source", "N_Dop Remote", "N_Dop Active": Value Change {
            n238 = event-data() -> ()  [unwired: 7 out]
            n239 = call "set_N_Dop.vi"("N_Dop Active"="N_Dop Active", "N_Dop Bubbler"="N_Dop Bubbler", "N_Dop H2 Dilute"="N_Dop H2 Dilute", "N_Dop Gas Source"="N_Dop Gas Source", "N_Dop Run"="N_Dop Run", "N_Dop Remote"="N_Dop Remote", "N_Dop Flow 4"="Set N Dopant Flow Rate 4", "N_Dop Flow 3"="Set N Dopant Flow Rate 3", "N_Dop Flow 2"="Set N Dopant Flow Rate 2", "N_Dop Flow 1"="Set N Dopant Flow Rate 1") -> ()  [unwired: 10 out]
            n240 = Number To Fractional String(number="Set N Dopant Flow Rate 2") -> (F-format string=w447:string)  [unwired: 3 in]
            n241 = Number To Fractional String(number="Set N Dopant Flow Rate 4") -> (F-format string=w419:string)  [unwired: 3 in]
            n242 = Number To Fractional String(number="Set N Dopant Flow Rate 1") -> (F-format string=w450:string)  [unwired: 3 in]
            n243 = Number To Fractional String(number="Set N Dopant Flow Rate 3") -> (F-format string=w444:string)  [unwired: 3 in]
            n244 = Select(t="N_Dop Active ", s="N_Dop Active", f="") -> (s? t:f=w427:string)
            n245 = Concatenate Strings("N_Dop Rate 2 " ("string"), w447, " " ("string")) -> (w429:string)
            n246 = Concatenate Strings("N_Dop Rate 4 " ("string"), w419, " " ("string")) -> (w418:string)
            n247 = Select(t="N_Dop Bubbler ", s="N_Dop Bubbler", f="") -> (s? t:f=w426:string)
            n248 = Concatenate Strings("N_Dop Rate 1 " ("string"), w450, " " ("string")) -> (w430:string)
            n249 = Select(t="N_Dop Run ", s="N_Dop Run", f="") -> (s? t:f=w425:string)
            n250 = Select(t="N_Dop Remote ", s="N_Dop Remote", f="") -> (s? t:f=w424:string)
            n251 = Select(t="N_Dop Gas Source ", s="N_Dop Gas Source", f="") -> (s? t:f=w423:string)
            n252 = Concatenate Strings("N_Dop Rate 3 " ("string"), w444, " " ("string")) -> (w428:string)
            n253 = global read "globals.vi" "Log String"() -> (w431:string)
            n254 = Concatenate Strings(w431, w430, w429, w428, w418, w427, w426, w425, w424, w423, "\r\n") -> (w421:string)
            n255 = global write "globals.vi" "Log String"(w421) -> ()
          }
          event "Display N or P": Value Change {
            n256 = event-data() -> ()  [unwired: 7 out]
            n257 = call "set_NP_Display.vi"("N/P Dopant DA Switch"="Display N or P") -> ()
          }
          event "Vac Remote", "Vac Exhaust", "Atm Exhaust": Value Change {
            n258 = event-data() -> ()  [unwired: 7 out]
            n259 = call "set_vacuum.vi"("Vac Remote"="Vac Remote", "Atm Exhaust"="Atm Exhaust", "Vac Exhaust"="Vac Exhaust") -> ()
            n260 = Select(t="Vac Exhaust ", s="Vac Exhaust", f="") -> (s? t:f=w456:string)
            n261 = Select(t="Atm Exhaust ", s="Atm Exhaust", f="") -> (s? t:f=w455:string)
            n262 = Select(t="Vac Remote ", s="Vac Remote", f="") -> (s? t:f=w454:string)
            n263 = global read "globals.vi" "Log String"() -> (w467:string)
            n264 = Concatenate Strings(w467, w456, w455, w454, "\r\n") -> (w466:string)
            n265 = global write "globals.vi" "Log String"(w466) -> ()
          }
        }
      }
    }
  }
